vi "Macro Array_Text interchange.vi"(7 "Command":enum16{"Array to Text", "Text to Array"}(ring), 8 "error in (no error)":errorcluster, 10 "Macro Text IN":string, 11 "Macro Array IN":string[](array[string])) -> (0 "error out":errorcluster, 2 "Macro Text OUT":string, 3 "Macro Array OUT":string[](array[string]))   [LabVIEW 2012]
doc: "SciScan 1.2 160622"
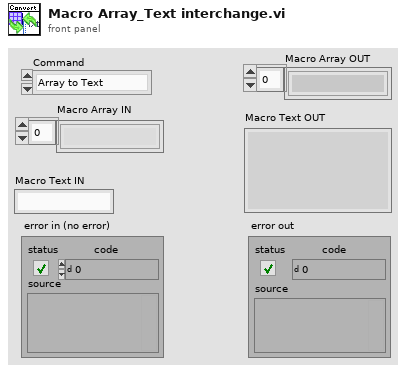
[diagram p1: front panel]
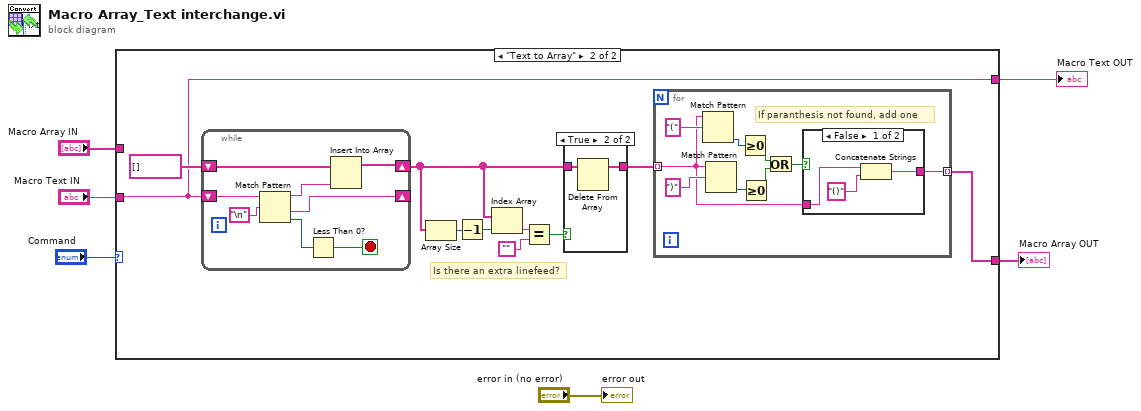
[diagram p0: block diagram]
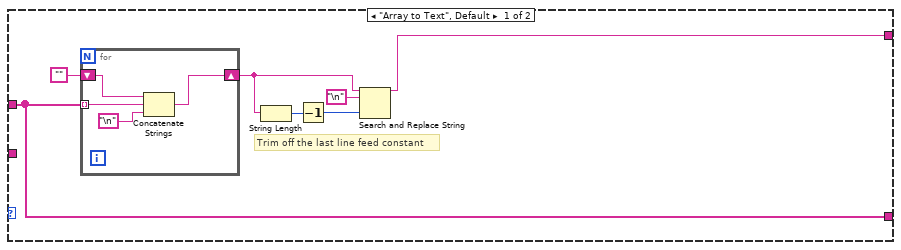
[diagram p2: hidden frame]
diagram:
  n1 = case shown="\"Text to Array\"" "Command" {
    tunnel: [w12 w19] -> w5
    tunnel: "Macro Text IN" -> [_ w18]
    tunnel: "Macro Array IN" -> [w12 _]
    tunnel: [w7 w18] -> w2
    frame "Array to Text", Default {
      # "Trim off the last line feed constant"
      n2 = for {
        tunnel: w12 -> [w17] mode=indexing
        shift-right: [w14] -> w9
        shift-left: "" -> [w15]
        n3 = Concatenate Strings(w15, w17, "\n") -> (w14:string)
      }
      n4 = String Length(string=w9) -> (length=w11:i32)
      n5 = Decrement(x=w11) -> (x-1=w10:i32)
      n6 = Search and Replace String(input string=w9, search string="\n", offset=w10) -> (result string=w7:string)  [unwired: 5 in, 3 out]
    }
    frame "Text to Array" {
      # "Is there an extra linefeed?"
      n7 = while {
        shift-right: [w44] -> w24
        shift-left: string[] [] -> [w48]
        shift-right: [w45] -> _
        shift-left: w18 -> [w47]
        stop <- w49 stop-if-true
        n8 = Match Pattern(string=w47, regular expression="\n") -> (before substring=w46:string, after substring=w45:string, offset past match=w50:i32)  [unwired: 1 in, 1 out]
        n9 = Less Than 0?(x=w50) -> (x < 0?=w49:bool)
        n10 = Insert Into Array(array=w48, new element=w46) -> (w44:string[])  [unwired: 1 in]
      }
      n11 = Array Size(array=w24) -> (size(s)=w26:i32)
      n12 = Decrement(x=w26) -> (x-1=w25:i32)
      n13 = Index Array(array=w24, index=w25) -> (element=w23:string)
      n14 = Equal?(x=w23, y="") -> (x = y?=w21:bool)
      n15 = case shown="True" w21 {
        tunnel: [w41 w43] -> w20
        tunnel: w24 -> [w41 w42]
        frame False {
        }
        frame True {
          n16 = Delete From Array(array=w42) -> (array with subset deleted=w43:string[])  [unwired: 2 in, 1 out]
        }
      }
      n17 = for {
        tunnel: w20 -> [w29] mode=indexing
        tunnel: [w28] -> w19 mode=indexing
        # "If paranthesis not found, add one"
        n18 = Match Pattern(string=w29, regular expression="(") -> (offset past match=w34:i32)  [unwired: 1 in, 3 out]
        n19 = Match Pattern(string=w29, regular expression=")" ("string")) -> (offset past match=w35:i32)  [unwired: 1 in, 3 out]
        n20 = Greater Or Equal To 0?(x=w34) -> (x >= 0?=w33:bool)
        n21 = Greater Or Equal To 0?(x=w35) -> (x >= 0?=w32:bool)
        n22 = Or(x=w33, y=w32) -> (x .or. y?=w31:bool)
        n23 = case shown="False" w31 {
          tunnel: w29 -> [w39 w40]
          tunnel: [w37 w40] -> w28
          frame False {
            n24 = Concatenate Strings(w39, "()" ("string")) -> (w37:string)
          }
          frame True {
          }
        }
      }
    }
  }
  "Macro Text OUT" <- w2
  "Macro Array OUT" <- w5
  "error out" <- "error in (no error)"
